vi "DecimatedCycle.vi"(9 "Reset Cycle":bool caption="Reset Cycle (F)", 10 "n":i32) -> (2 "Decimated Cycle":i32, 4 "Falling Edge":bool, 5 "Rising Edge":bool)   [LabVIEW 2017, in "GPNumeric.lvlib"]
doc: "Outputs a <B>Decimated Cycle</B> when called repeatedly.\n\nThe <B>Decimated Cycle</B> will count up from 0 at a rate <B>n</B> times slower than the calling rate.\n\nWhen a new decimated period starts <B>Rising Edge</B> will be True, else it will be False. When a decimated period ends <B>Falling Edge</B> will be True, else it will be False. This can be useful when you want to execute some code only at each n'th iteration of a loop for instance.\n\nIf you run this VI enough times <B>Decimated Cycle</B> will eventually latch at I32 max, but <B>Rising Edge</B> and <B>Falling Edge</B> will continue forever to change with the proper decimation.\n\nSetting <B>Reset Cycle</B> to True makes <B>Cycle</B> start from 0 again.\n\nThis VI is inlined.\n\nSteen Schmidt\nGPower\n7/4 2014"
uses:
  GPNumeric.lvlib
panel:
  # "Copyright © 2014\nGPower\nSee enclosed license file for terms and conditions"
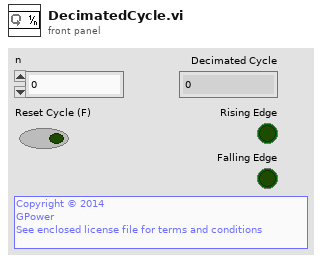
[diagram p1: front panel]
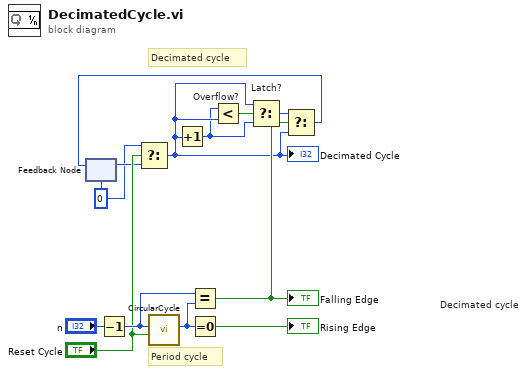
[diagram p0: block diagram]
diagram:
  w1 = 0
  # "Period cycle"
  # "Decimated cycle"
  n1 = feedback #1 "Decimated cycle"(w1) -> (w6:i32)
  n2 = Decrement(x="n") -> (x-1=w10:i32)
  n3 = Select(t=w1, s="Reset Cycle", f=w6) -> (s? t:f=w4:i32)
  "Decimated Cycle" <- w4
  n4 = call "CircularCycle.vi"("Reset Cycle"="Reset Cycle", "n"=w10) -> ("Circular Cycle"=w11:i32)  [unwired: 9 in]
  n5 = Increment(x=w4) -> (x+1=w3:i32)
  n6 = Equal?(x=w10, y=w11) -> (x = y?=w9:bool)
  "Falling Edge" <- w9
  n7 = Equal To 0?(x=w11) -> (x = 0?=→"Rising Edge":bool)
  n8 = Less? "Overflow?"(x=w3, y=w4) -> (x < y?=w5:bool)
  n9 = Select "Latch?"(t=w4, s=w5, f=w3) -> (s? t:f=w2:i32)
  n10 = Select(t=w2, s=w9, f=w4) -> (s? t:f=w8:i32)
  n11 = feedback-in #1(w8) -> ()
